vi "Find External Path Combinations.vi"(11 "Found Common Paths in":string[](array[string])) -> (3 "External Path Combinations":string[](array[string]))   [LabVIEW 2019, in "Project.Dependencies Finder.lvlib"]
doc: "Find valid folder names and combinations of up to two names from given paths."
uses:
  Project.Dependencies Finder.lvlib
  87b231cf-aae6-4cc0-9b38-4f8b959dfd4e.vi
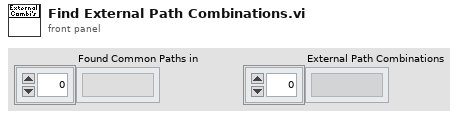
[diagram p1: front panel]
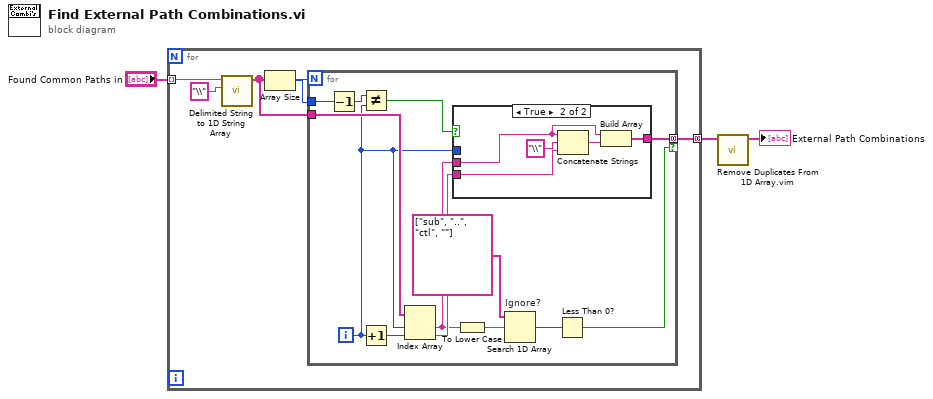
[diagram p0: block diagram]
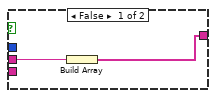
[diagram p2: hidden frame]
diagram:
  n1 = for {
    tunnel: "Found Common Paths in" -> [w7] mode=indexing
    tunnel: [w4] -> w2 mode=concatenating
    n2 = call <vilib>:"Delimited String to 1D String Array.vi"("delimiter"="\\" ("search string"), "delimited string"=w7) -> ("string array"=w6:string[])  [unwired: 9 in]
    n3 = Array Size(array=w6) -> (size(s)=w5:i32)
    n4 = for {
      N: w5 -> [_]
      tunnel: w6 -> [w17]
      tunnel: w5 -> [w21]
      tunnel: [w18] -> w4 mode=concatenating if=w10
      i -> [w16]
      n5 = Decrement(x=w21) -> (x-1=w20:i32)
      n6 = Not Equal?(x=w20, y=w16) -> (x != y?=w19:bool)
      n7 = Increment(x=w16) -> (x+1=w15:i32)
      n8 = Index Array(array=w17, index #1=w16, index #2=w15) -> (element #1=w13:string, element #2=w14:string)
      n9 = case shown="True" w19 {
        tunnel: w16 -> [_ _]
        tunnel: [w23 w26] -> w18
        tunnel: w13 -> [w22 w25]
        tunnel: w14 -> [_ w24]
        frame False {
          n10 = Build Array(w22) -> (w23:string[])
        }
        frame True {
          n11 = Concatenate Strings(w25, "\\" ("search string"), w24) -> (w27:string)
          n12 = Build Array(w25, w27) -> (w26:string[])
        }
      }
      n13 = To Lower Case(string=w13) -> (all lower case string=w12:string)
      n14 = Search 1D Array "Ignore?"(1D array=string[] ["sub", "..", "ctl", ""], element=w12) -> (index of element=w11:i32)  [unwired: 1 in]
      n15 = Less Than 0?(x=w11) -> (x < 0?=w10:bool)
    }
  }
  n16 = call "Remove Duplicates From 1D Array.vim"("array"=w2) -> ("array with duplicates removed"=→"External Path Combinations":string[])  [unwired: 10 in]
